vi "TSLIN_Queue_Quit.vi"(8 "error in (no error)":errorcluster caption="错误输入（无错误）", 10 "receiver":string, 11 "Channels used":u16) -> (0 "error out":errorcluster caption="错误输出")   [LabVIEW 2014]
uses:
  <vilib>/Utility/miscctls.llb/LVPointTypeDef.ctl
panel:
  out "Exiting...":u8(slide) scale=0.0..100.0
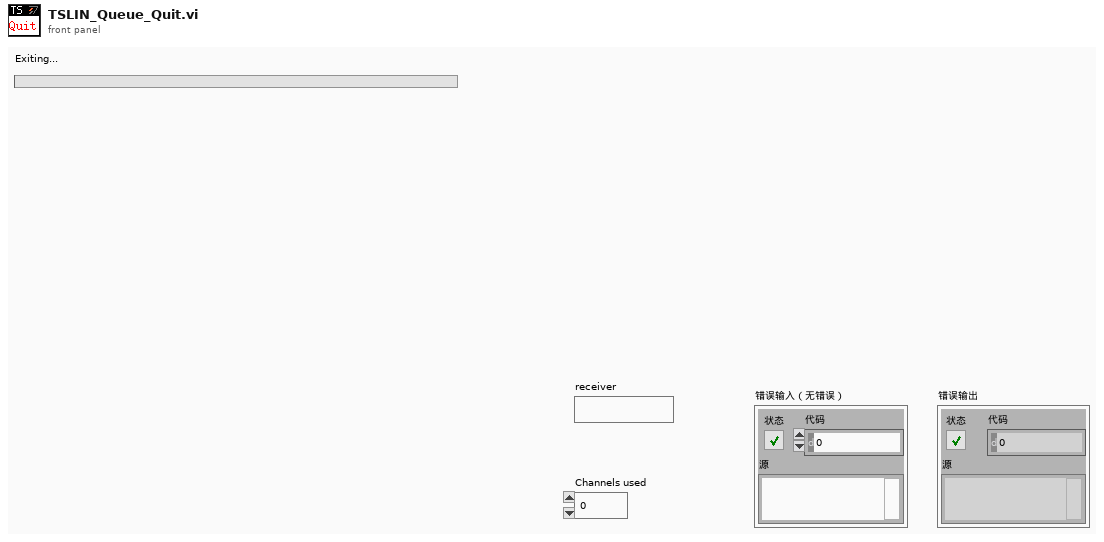
[diagram p1: front panel]
types:
  T1 = typedef "LVPointTypeDef.ctl" = cluster{"Horizontal":i16, "Vertical":i16}
  T2 = cluster{"Sender":string, "receiver":string, "message":string, "data":variant}
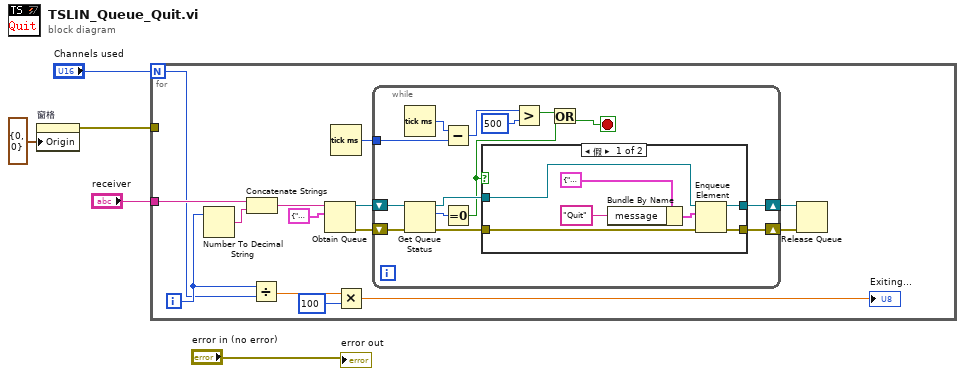
[diagram p0: block diagram]
diagram:
  n1 = property on="窗格" class="Pane"("Origin"=T1 {"Horizontal"=0, "Vertical"=0} ("原点")) -> (error out=w2:errorcluster)  [unwired: 2 in, 1 out]
  n2 = for {
    N: "Channels used" -> [w6]
    tunnel: "receiver" -> [w14]
    tunnel: w2 -> [_]
    i -> [w7]
    n3 = Number To Decimal String(number=w7) -> (decimal integer string=w15:string)  [unwired: 1 in]
    n4 = Concatenate Strings(w14, w15) -> (w13:string)
    n5 = Divide(x=w7, y=w6) -> (x/y=w10:dbl)
    n6 = Obtain Queue(name (unnamed)=w13, element data type=T2 {"Sender"="", "receiver"="", "message"="", "data"=variant} ("Communication message")) -> (queue out=w19:refnum<queue>, error out=w17:errorcluster)  [unwired: 3 in, 1 out]
    n7 = Tick Count (ms)() -> (millisecond timer value=w11:u32)
    n8 = Multiply(x=w10, y=u8 100) -> (x*y=→"Exiting...":dbl)
    n9 = while {
      shift-right: [w33] -> w18
      shift-left: w19 -> [w25]
      shift-right: [w32] -> w16
      shift-left: w17 -> [w27]
      tunnel: w11 -> [w30]
      stop <- w21 stop-if-true
      n10 = Tick Count (ms)() -> (millisecond timer value=w31:u32)
      n11 = Get Queue Status(queue=w25, error in (no error)=w27) -> (queue out=w24:refnum<queue>, # pending remove=w23:i32, error out=w26:errorcluster)  [unwired: 1 in, 5 out]
      n12 = Subtract(x=w31, y=w30) -> (x-y=w29:u32)
      n13 = Equal To 0?(x=w23) -> (x = 0?=w22:bool)
      n14 = case shown="假" w22 {
        tunnel: [w40 w42] -> w33
        tunnel: [w39 w41] -> w32
        tunnel: w26 -> [w35 w41]
        tunnel: w24 -> [w34 w42]
        frame False {
          n15 = Bundle By Name(cluster=T2 {"Sender"="", "receiver"="", "message"="Quit", "data"=variant} ("元素"), "message"="Quit") -> (w37:T2)
          n16 = Enqueue Element(queue=w34, element=w37, error in (no error)=w35) -> (queue out=w40:refnum<queue>, error out=w39:errorcluster)  [unwired: 1 in, 1 out]
        }
        frame True {
        }
      }
      n17 = Greater?(x=w29, y=u32 500) -> (0:w20:bool)
      n18 = Or(x=w20, y=w22) -> (x .or. y?=w21:bool)
    }
    n19 = Release Queue(queue=w18, error in (no error)=w16) -> ()  [unwired: 1 in, 3 out]
  }
  "error out" <- "error in (no error)"
